vi "Write Root Lifetime.vi"(10 "Root Lifetime":T1, 11 "Base Actor in":refnum<class "Base Actor.lvclass">) -> (3 "Base Actor out":refnum<class "Base Actor.lvclass">)   [LabVIEW 2020, in "jettl.lvlib" / "Base jettl Actor.lvlib" / "Base Actor.lvlib" / "Base Actor.lvclass"]
uses:
  Base Actor.lvclass
  Base Actor.lvclass/Base Actor.ctl
  Actor/Actor.lvclass
  Root Lifetime.ctl
  jettl.lvlib
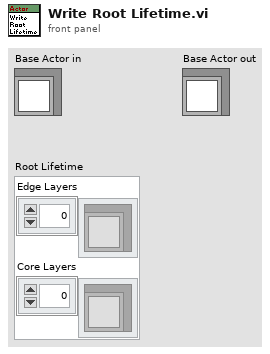
[diagram p1: front panel]
types:
  T1 = typedef "jettl.lvlib/Root Lifetime.ctl" = cluster{"Edge Layers":refnum<class "Actor.lvclass">[], "Core Layers":refnum<class "Actor.lvclass">[]}
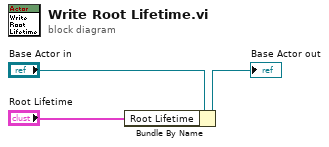
[diagram p0: block diagram]
diagram:
  n1 = Bundle By Name(cluster="Base Actor in", "Root Lifetime"="Root Lifetime") -> (→"Base Actor out":refnum<class "Base Actor.lvclass">)
